vi "AK Amium Auswerten.vi"(8 "Verknüpfter String":string, 9 "ATEM Index":string[](array[string]), 10 "Array":string[](array[string])) -> ()   [LabVIEW 2020, in "Amium PNS.lvlib" / "AK Kommunikation.lvlib"]
uses:
  AK Kommunikation.lvlib
  Aktion FGV Amium Daten.ctl
  Amium Kommandos verwalten Aktionen.ctl
  Amium Zustand.ctl
  Amium ErrorCluster.ctl
  Amium PNS.lvlib
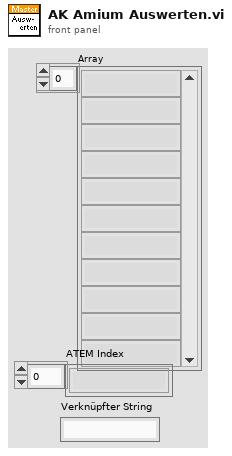
[diagram p1: front panel]
types:
  T1 = typedef "Amium PNS.lvlib/Aktion FGV Amium Daten.ctl" = enum16{"lesen", "Komm Daten", "Daten", "Error", "Regler", "Grenzwerte", "laden", "speichern"}
  T2 = typedef "Amium PNS.lvlib/AK Kommunikation.lvlib/Amium Kommandos verwalten Aktionen.ctl" = enum16{"lesen", "setzen Ende", "setzen Pos1", "senden", "initalisieren", "prüfen", "Kommandos"}
  T3 = typedef "Amium PNS.lvlib/Amium ErrorCluster.ctl" = cluster{"Messgasdruck":bool, "Temperatur":bool, "Steuerluft":bool, "Temperatur HL 1":bool, "Temperatur HL 2":bool, "Temperatur HL 3":bool, "Temperatur HL 4":bool, "Temperatur HL 5":bool, "Temperatur HL 6":bool, "Temperatur HL 7":bool, "Temperatur HL 8":bool, "Temperatur HL 9":bool, "Temperatur HL 10":bool, "Temperatur 11 Ofen MGF/Filter":bool, "Temperatur HL12":bool, "Temperatur 13 Ofen MGP/Pumpe":bool, "Temperatur HL 14":bool}
  T4 = typedef "Amium PNS.lvlib/Daten Cluster.ctl" = cluster{"Amium Zustände":T5, "Samplepoint am PNS":i16, "Gerätekennung":string, "aktiver Samplepoint":i16[], "Messgasdruck":sgl}
  T5 = typedef "Amium PNS.lvlib/Amium Zustand.ctl" = u16
  T6 = typedef "Amium PNS.lvlib/Temperaturregler Cluster.ctl" = cluster{"Istwert":sgl, "Sollwert":sgl, "Stellgröße":sgl, "Status":sgl, "Error":sgl}
  T7 = typedef "Amium PNS.lvlib/Amium Anlagengrenzwerte PNS.ctl" = cluster{"Filter:":T8, "Ventilplatte:":T8, "Heizleitung 1:":T8, "Heizleitung 2:":T8, "Heizleitung 3:":T8, "Heizleitung 4:":T8, "Heizleitung 5:":T8, "Heizleitung 6:":T8, "Heizleitung 7:":T8, "Heizleitung 8:":T8, "Heizleitung 9:":T8, "Heizleitung 10:":T8, "Heizleitung 11:":T8, "Heizleitung 12:":T8}
  T8 = typedef "Amium PNS.lvlib/Amium Anlagengrenzwerte-Parameter Anzeige.ctl" = cluster{"Sollwert":T9, "Warn-Min":T9, "Warn-Max":T9, "Abschalt-Min":T9, "Abschalt-Max":T9, "Regler":u16}
  T9 = typedef "Zahlen-Eingabefeld.ctl" = sgl
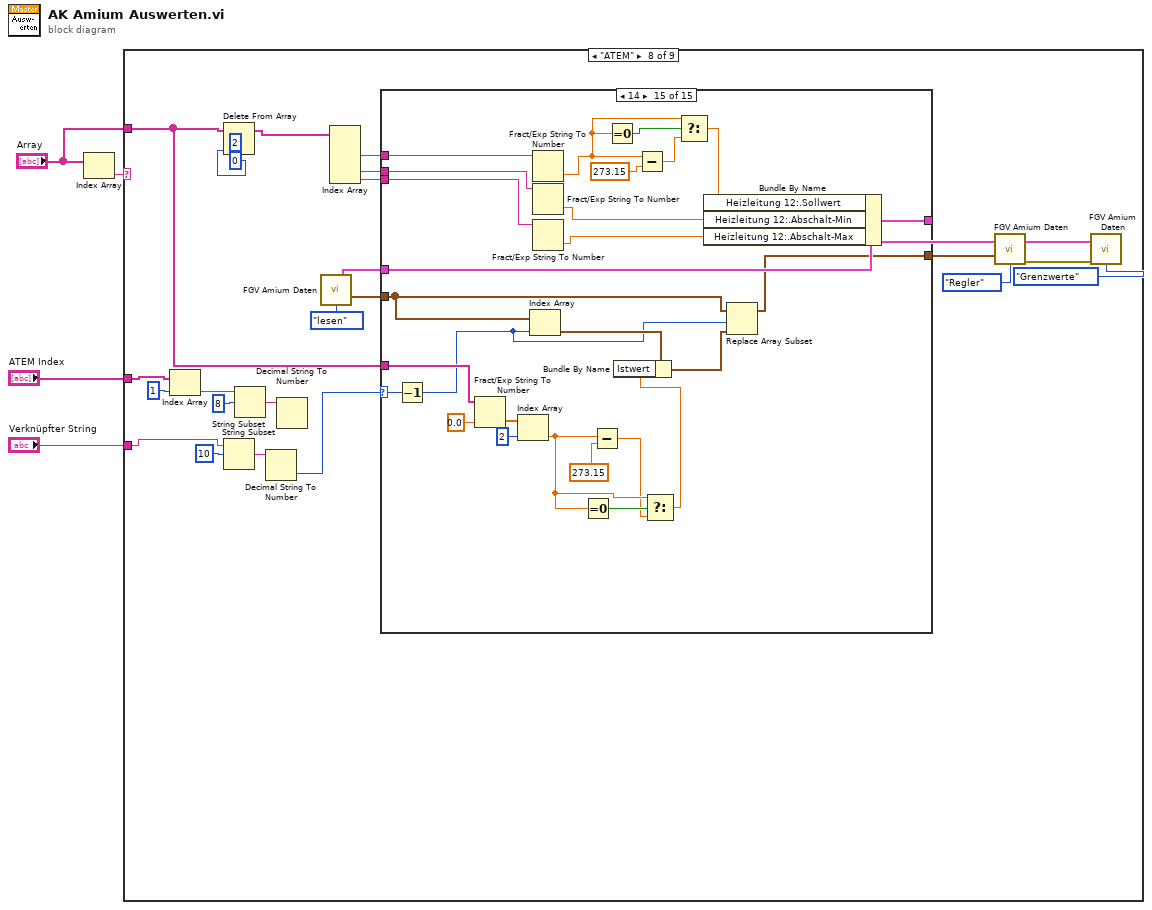
[diagram p0: block diagram]
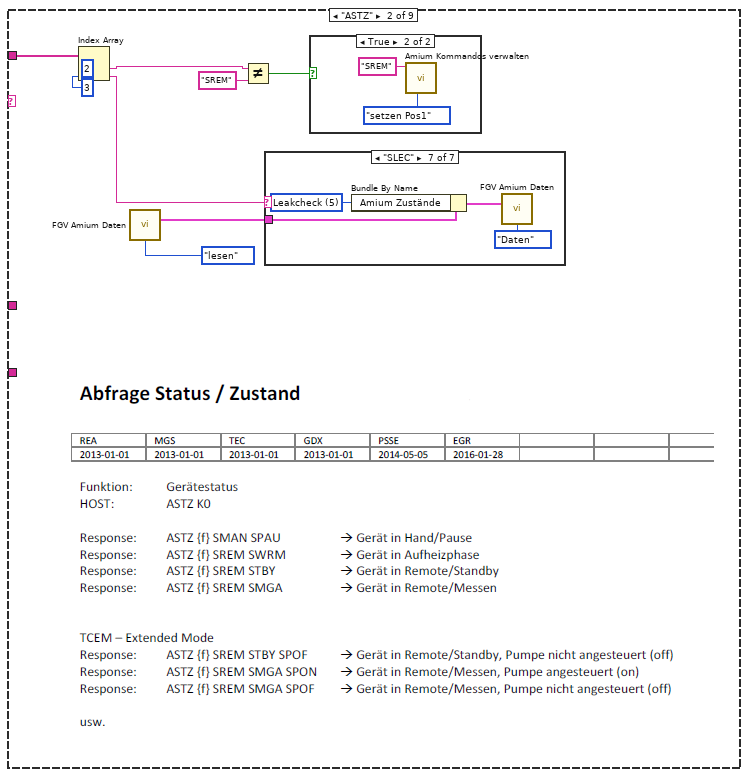
[diagram p3: hidden frame]
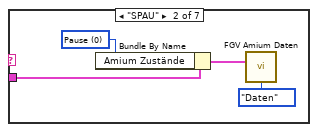
[diagram p5: hidden frame]
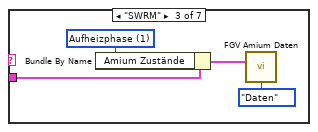
[diagram p6: hidden frame]
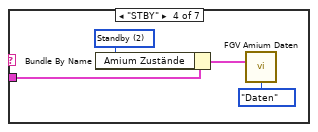
[diagram p7: hidden frame]
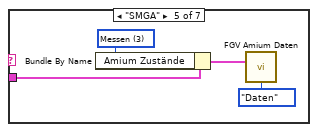
[diagram p8: hidden frame]
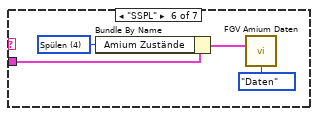
[diagram p9: hidden frame]
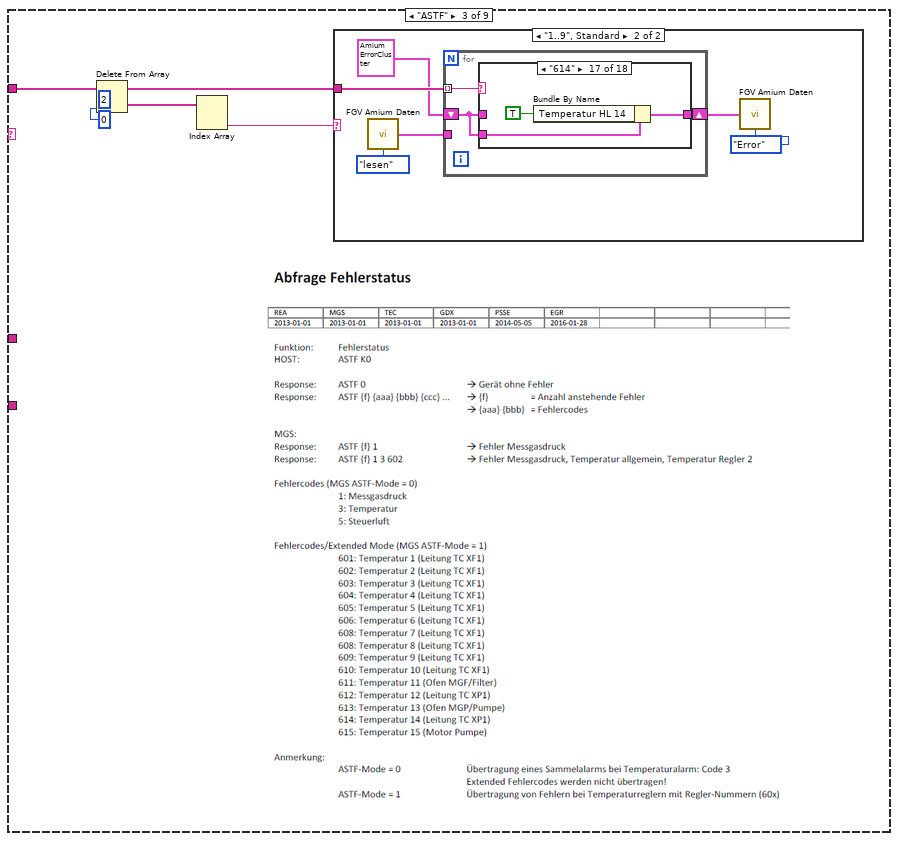
[diagram p11: hidden frame]
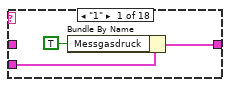
[diagram p13: hidden frame]
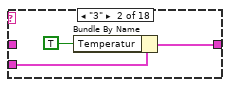
[diagram p14: hidden frame]
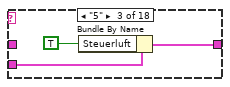
[diagram p15: hidden frame]
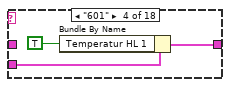
[diagram p16: hidden frame]
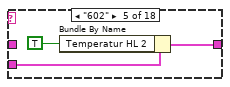
[diagram p17: hidden frame]
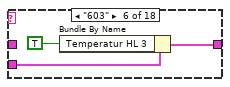
[diagram p18: hidden frame]
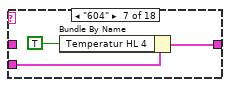
[diagram p19: hidden frame]
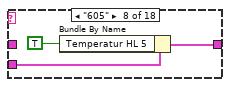
[diagram p20: hidden frame]
diagram:
  n1 = Index Array(array="Array") -> (element=w4:string)  [unwired: 1 in]
  n2 = case shown="\"ATEM\"" w4 {
    tunnel: "Array" -> [_ w13 w45 w115 w122 w136 w170 w180 w588]
    tunnel: "ATEM Index" -> [_ _ _ _ _ _ _ w185 _]
    tunnel: "Verknüpfter String" -> [_ _ _ _ _ w124 _ w184 _]
    frame "False", Default {
    }
    frame "ASTZ" {
      n3 = Index Array(array=w13, index #1=2 ("Index"), index #2=3 ("Index")) -> (element #1=w10:string, element #2=w7:string)
      n4 = call "FGV Amium Daten.vi"("Aktion"=Aktion_FGV_Amium_Daten."lesen") -> ("Amium Daten"=w5:T4)  [unwired: 9 in, 5 out]
      n5 = Not Equal?(x=w10, y="SREM" ("neues Kommando")) -> (x != y?=w9:bool)
      n6 = case shown="\"SLEC\"" w7 {
        tunnel: w5 -> [_ w17 w21 w25 w29 w33 w37]
        frame "False", Default {
        }
        frame "SPAU" {
          w16 = T5 0 items=["Pause", "Aufheizphase", "Standby", "Messen"] ("Amium Zustände")
          n7 = Bundle By Name(cluster=w17, "Amium Zustände"=w16) -> (w14:T4)
          n8 = call "FGV Amium Daten.vi"("Amium Daten"=w14, "Aktion"=Aktion_FGV_Amium_Daten."Daten") -> ()  [unwired: 8 in, 6 out]
        }
        frame "SWRM" {
          w20 = T5 1 items=["Pause", "Aufheizphase", "Standby", "Messen"] ("Amium Zustände")
          n9 = Bundle By Name(cluster=w21, "Amium Zustände"=w20) -> (w18:T4)
          n10 = call "FGV Amium Daten.vi"("Amium Daten"=w18, "Aktion"=Aktion_FGV_Amium_Daten."Daten") -> ()  [unwired: 8 in, 6 out]
        }
        frame "STBY" {
          w24 = T5 2 items=["Pause", "Aufheizphase", "Standby", "Messen"] ("Amium Zustände")
          n11 = Bundle By Name(cluster=w25, "Amium Zustände"=w24) -> (w22:T4)
          n12 = call "FGV Amium Daten.vi"("Amium Daten"=w22, "Aktion"=Aktion_FGV_Amium_Daten."Daten") -> ()  [unwired: 8 in, 6 out]
        }
        frame "SMGA" {
          w28 = T5 3 items=["Pause", "Aufheizphase", "Standby", "Messen"] ("Amium Zustände")
          n13 = Bundle By Name(cluster=w29, "Amium Zustände"=w28) -> (w26:T4)
          n14 = call "FGV Amium Daten.vi"("Amium Daten"=w26, "Aktion"=Aktion_FGV_Amium_Daten."Daten") -> ()  [unwired: 8 in, 6 out]
        }
        frame "SSPL" {
          w30 = T5 4 items=["Pause", "Aufheizphase", "Standby", "Messen", "Spülen"] ("Amium Zustände")
          n15 = Bundle By Name(cluster=w33, "Amium Zustände"=w30) -> (w31:T4)
          n16 = call "FGV Amium Daten.vi"("Amium Daten"=w31, "Aktion"=Aktion_FGV_Amium_Daten."Daten") -> ()  [unwired: 8 in, 6 out]
        }
        frame "SLEC" {
          w34 = T5 5 items=["Pause", "Aufheizphase", "Standby", "Messen", "Spülen", "Leakcheck"] ("Amium Zustände")
          n17 = Bundle By Name(cluster=w37, "Amium Zustände"=w34) -> (w35:T4)
          n18 = call "FGV Amium Daten.vi"("Amium Daten"=w35, "Aktion"=Aktion_FGV_Amium_Daten."Daten") -> ()  [unwired: 8 in, 6 out]
        }
      }
      n19 = case shown="True" w9 {
        frame False {
        }
        frame True {
          n20 = call "Amium Kommandos verwalten.vi"("Aktionen"=Amium_Kommandos_verwalten_Aktionen."setzen Pos1", "neues Kommando"="SREM") -> ()  [unwired: 7 in, 3 out]
        }
      }
    }
    frame "ASTF" {
      n21 = Delete From Array(array=w45, length=2 ("Länge"), index=0 ("Index")) -> (deleted portion=w41:string[], array with subset deleted=w42:string[])
      n22 = Index Array(array=w41) -> (element #2=w40:string)  [unwired: 2 in, 1 out]
      n23 = case shown="\"1..9\", Standard" w40 {
        tunnel: w42 -> [_ w51]
        frame "0" {
        }
        frame "1..9", Default {
          n24 = call "FGV Amium Daten.vi"("Aktion"=Aktion_FGV_Amium_Daten."lesen") -> ("Fehler Cluster"=w47:T3)  [unwired: 9 in, 5 out]
          n25 = for {
            tunnel: w51 -> [w54] mode=indexing
            shift-right: [w53] -> w48
            shift-left: T3 {"Messgasdruck"=FALSE, "Temperatur"=FALSE, "Steuerluft"=FALSE, "Temperatur HL 1"=FALSE, "Temperatur HL 2"=FALSE, "Temperatur HL 3"=FALSE, "Temperatur HL 4"=FALSE, "Temperatur HL 5"=FALSE, "Temperatur HL 6"=FALSE, "Temperatur HL 7"=FALSE, "Temperatur HL 8"=FALSE, "Temperatur HL 9"=FALSE, "Temperatur HL 10"=FALSE, "Temperatur 11 Ofen MGF/Filter"=FALSE, "Temperatur HL12"=FALSE, "Temperatur 13 Ofen MGP/Pumpe"=FALSE, "Temperatur HL 14"=FALSE} ("Fehler Cluster") -> [w52]
            tunnel: w47 -> [_]
            n26 = case shown="\"614\"" w54 {
              tunnel: w52 -> [w57 w60 w63 w66 w69 w72 w75 w78 w81 w84 w87 w90 w93 w96 w99 w102 w105 _]
              tunnel: [w55 w58 w61 w64 w67 w70 w73 w76 w79 w82 w85 w88 w91 w94 w97 w100 w103 w106] -> w53
              tunnel: w52 -> [_ _ _ _ _ _ _ _ _ _ _ _ _ _ _ _ _ w106]
              frame "1" {
                n27 = Bundle By Name(cluster=w57, "Messgasdruck"=TRUE) -> (w55:T3)
              }
              frame "3" {
                n28 = Bundle By Name(cluster=w60, "Temperatur"=TRUE ("Messgasdruck")) -> (w58:T3)
              }
              frame "5" {
                n29 = Bundle By Name(cluster=w63, "Steuerluft"=TRUE ("Messgasdruck")) -> (w61:T3)
              }
              frame "601" {
                n30 = Bundle By Name(cluster=w66, "Temperatur HL 1"=TRUE ("Messgasdruck")) -> (w64:T3)
              }
              frame "602" {
                n31 = Bundle By Name(cluster=w69, "Temperatur HL 2"=TRUE ("Messgasdruck")) -> (w67:T3)
              }
              frame "603" {
                n32 = Bundle By Name(cluster=w72, "Temperatur HL 3"=TRUE ("Messgasdruck")) -> (w70:T3)
              }
              frame "604" {
                n33 = Bundle By Name(cluster=w75, "Temperatur HL 4"=TRUE ("Messgasdruck")) -> (w73:T3)
              }
              frame "605" {
                n34 = Bundle By Name(cluster=w78, "Temperatur HL 5"=TRUE ("Messgasdruck")) -> (w76:T3)
              }
              frame "606" {
                n35 = Bundle By Name(cluster=w81, "Temperatur HL 6"=TRUE ("Messgasdruck")) -> (w79:T3)
              }
              frame "607" {
                n36 = Bundle By Name(cluster=w84, "Temperatur HL 7"=TRUE ("Messgasdruck")) -> (w82:T3)
              }
              frame "608" {
                n37 = Bundle By Name(cluster=w87, "Temperatur HL 8"=TRUE ("Messgasdruck")) -> (w85:T3)
              }
              frame "609" {
                n38 = Bundle By Name(cluster=w90, "Temperatur HL 9"=TRUE ("Messgasdruck")) -> (w88:T3)
              }
              frame "610" {
                n39 = Bundle By Name(cluster=w93, "Temperatur HL 10"=TRUE ("Messgasdruck")) -> (w91:T3)
              }
              frame "611" {
                n40 = Bundle By Name(cluster=w96, "Temperatur 11 Ofen MGF/Filter"=TRUE ("Messgasdruck")) -> (w94:T3)
              }
              frame "612" {
                n41 = Bundle By Name(cluster=w99, "Temperatur HL12"=TRUE ("Messgasdruck")) -> (w97:T3)
              }
              frame "613" {
                n42 = Bundle By Name(cluster=w102, "Temperatur 13 Ofen MGP/Pumpe"=TRUE ("Messgasdruck")) -> (w100:T3)
              }
              frame "614" {
                n43 = Bundle By Name(cluster=w105, "Temperatur HL 14"=TRUE ("Messgasdruck")) -> (w103:T3)
              }
              frame "0", Default {
              }
            }
          }
          n44 = call "FGV Amium Daten.vi"("Fehler Cluster"=w48, "Aktion"=Aktion_FGV_Amium_Daten."Error") -> ()  [unwired: 8 in, 6 out]
        }
      }
    }
    frame "ACFG" {
      n45 = Index Array(array=w115, index=2 ("Index")) -> (element=w113:string)
      n46 = Decimal String To Number(string=w113, default (0L)=i16 0 ("Samplepoint am PNS")) -> (number=w110:i16)  [unwired: 1 in, 1 out]
      n47 = call "FGV Amium Daten.vi"("Aktion"=Aktion_FGV_Amium_Daten."lesen") -> ("Amium Daten"=w111:T4)  [unwired: 9 in, 5 out]
      n48 = Bundle By Name(cluster=w111, "Samplepoint am PNS"=w110) -> (w107:T4)
      n49 = call "FGV Amium Daten.vi"("Amium Daten"=w107, "Aktion"=Aktion_FGV_Amium_Daten."Daten") -> ()  [unwired: 8 in, 6 out]
    }
    frame "AKEN" {
      n50 = Index Array(array=w122, index=2 ("Index")) -> (element=w116:string)
      n51 = call "FGV Amium Daten.vi"("Aktion"=Aktion_FGV_Amium_Daten."lesen") -> ("Amium Daten"=w119:T4)  [unwired: 9 in, 5 out]
      n52 = Bundle By Name(cluster=w119, "Gerätekennung"=w116) -> (w117:T4)
      n53 = call "FGV Amium Daten.vi"("Amium Daten"=w117, "Aktion"=Aktion_FGV_Amium_Daten."Daten") -> ()  [unwired: 8 in, 6 out]
    }
    frame "ATES" {
      n54 = String Subset(string=w124, offset (0)=10 ("Offset (0)")) -> (substring=w126:string)  [unwired: 1 in]
      n55 = Delete From Array(array=w136, length=2 ("Länge"), index=0 ("Index")) -> (array with subset deleted=w131:string[])  [unwired: 1 out]
      n56 = Decimal String To Number(string=w126) -> (number=w123:i32)  [unwired: 2 in, 1 out]
      n57 = Array Size(array=w131) -> (size(s)=w130:i32)
      n58 = Fract/Exp String To Number(string=w131, default (0 dbl)=sgl 0.0) -> (number=w132:sgl[])  [unwired: 2 in, 1 out]
      n59 = To Double Precision Float(number=w130) -> (double precision float=w127:dbl)
      n60 = Divide(x=w127, y=5.0) -> (x/y=w128:dbl)
      n61 = To Long Integer(number=w128) -> ()  [unwired: 1 out]
      n62 = case shown="0..14, Standard" w123 {
        selector: w123 -> [_ w163]
        tunnel: w132 -> [w138 w154]
        frame 20 {
          n63 = for {
            N: 10 -> [_]
            shift-right: [w151] -> _
            shift-left: w138 -> [w152]
            tunnel: [w139] -> _
            i -> [w141]
            stop <- w150 stop-if-true
            n64 = Split 1D Array(array=w152, index=5 ("Index")) -> (first subarray=w148:sgl[], second subarray=w151:sgl[])
            n65 = Empty Array?(array=w151) -> (empty?=w150:bool)
            n66 = Index Array(array=w148, index=3 ("Index")) -> (element=w142:sgl)
            n67 = call "FGV Amium Daten.vi"("Aktion"=Aktion_FGV_Amium_Daten."lesen") -> ("Regler"=w145:T6[])  [unwired: 9 in, 5 out]
            n68 = Index Array(array=w145, index=w141) -> (element=w146:T6)
            n69 = Bundle By Name(cluster=w146, "Status"=w142) -> (w144:T6)
            n70 = Replace Array Subset(array=w145, new element=w144, index=w141) -> (w139:T6[])
            n71 = call "FGV Amium Daten.vi"("Regler"=w139, "Aktion"=Aktion_FGV_Amium_Daten."Regler") -> ()  [unwired: 8 in, 6 out]
          }
        }
        frame 0..14, Default {
          (unwired) 10
          n72 = Decrement(x=w163) -> (x-1=w153:i32)
          n73 = Index Array(array=w154, index=3 ("Index")) -> (element=w157:sgl)
          n74 = call "FGV Amium Daten.vi"("Aktion"=Aktion_FGV_Amium_Daten."lesen") -> ("Regler"=w160:T6[])  [unwired: 9 in, 5 out]
          n75 = Index Array(array=w160, index=w153) -> (element=w161:T6)
          n76 = Bundle By Name(cluster=w161, "Status"=w157) -> (w159:T6)
          n77 = Replace Array Subset(array=w160, new element=w159, index=w153) -> (w155:T6[])
          n78 = call "FGV Amium Daten.vi"("Regler"=w155, "Aktion"=Aktion_FGV_Amium_Daten."Regler") -> ()  [unwired: 8 in, 6 out]
        }
      }
    }
    frame "AENT" {
      n79 = Delete From Array(array=w170, length=2 ("Länge"), index=0 ("Index")) -> (array with subset deleted=w164:string[])  [unwired: 1 out]
      n80 = call "FGV Amium Daten.vi"("Aktion"=Aktion_FGV_Amium_Daten."lesen") -> ("Amium Daten"=w168:T4)  [unwired: 9 in, 5 out]
      n81 = for {
        tunnel: [w174] -> w167 mode=indexing
        tunnel: w164 -> [w173] mode=indexing
        n82 = Decimal String To Number(string=w173, default (0L)=i16 0 ("Samplepoint am PNS")) -> (number=w174:i16)  [unwired: 1 in, 1 out]
      }
      n83 = Bundle By Name(cluster=w168, "aktiver Samplepoint"=w167) -> (w165:T4)
      n84 = call "FGV Amium Daten.vi"("Amium Daten"=w165, "Aktion"=Aktion_FGV_Amium_Daten."Daten") -> ()  [unwired: 8 in, 6 out]
    }
    frame "ATEM" {
      n85 = Index Array(array=w185, index=1 ("Index")) -> (element=w187:string)
      n86 = Delete From Array(array=w180, length=2 ("Länge"), index=0 ("Index")) -> (array with subset deleted=w193:string[])  [unwired: 1 out]
      n87 = String Subset(string=w184, offset (0)=10 ("Offset (0)")) -> (substring=w183:string)  [unwired: 1 in]
      n88 = String Subset(string=w187, offset (0)=8 ("Offset (0)")) -> (substring=w194:string)  [unwired: 1 in]
      n89 = Decimal String To Number(string=w183) -> (number=w181:i32)  [unwired: 2 in, 1 out]
      n90 = Decimal String To Number(string=w194) -> ()  [unwired: 2 in, 2 out]
      n91 = call "FGV Amium Daten.vi"("Aktion"=Aktion_FGV_Amium_Daten."lesen") -> ("Grenzwerte PNS"=w196:T7, "Regler"=w176:T6[])  [unwired: 9 in, 4 out]
      n92 = Index Array(array=w193) -> (element #2=w192:string, element #4=w191:string, element #5=w190:string)  [unwired: 5 in, 2 out]
      n93 = case shown="14" w181 {
        selector: w181 -> [_ w219 w246 w273 w300 w327 w354 w381 w408 w435 w462 w489 w516 w543 w570]
        tunnel: w196 -> [w201 w228 w255 w282 w309 w336 w363 w390 w417 w444 w471 w498 w525 w552 w579]
        tunnel: w192 -> [_ w227 w254 w281 w308 w335 w362 w389 w416 w443 w470 w497 w524 w551 w578]
        tunnel: w191 -> [_ w226 w253 w280 w307 w334 w361 w388 w415 w442 w469 w496 w523 w550 w577]
        tunnel: w190 -> [_ w224 w251 w278 w305 w332 w359 w386 w413 w440 w467 w494 w521 w548 w575]
        tunnel: [w201 w222 w249 w276 w303 w330 w357 w384 w411 w438 w465 w492 w519 w546 w573] -> w188
        tunnel: w180 -> [_ w220 w247 w274 w301 w328 w355 w382 w409 w436 w463 w490 w517 w544 w571]
        tunnel: [w200 w212 w239 w266 w293 w320 w347 w374 w401 w428 w455 w482 w509 w536 w563] -> w178
        tunnel: w176 -> [w200 w214 w241 w268 w295 w322 w349 w376 w403 w430 w457 w484 w511 w538 w565]
        frame 0, Default {
        }
        frame 1 {
          n94 = Decrement(x=w219) -> (x-1=w213:i32)
          n95 = Fract/Exp String To Number(string=w220, default (0 dbl)=sgl 0.0) -> (number=w217:sgl[])  [unwired: 2 in, 1 out]
          n96 = Index Array(array=w217, index=2 ("Index")) -> (element=w204:sgl)
          n97 = Index Array(array=w214, index=w213) -> (element=w218:T6)
          n98 = Fract/Exp String To Number(string=w227) -> (number=w208:dbl)  [unwired: 3 in, 1 out]
          n99 = Fract/Exp String To Number(string=w226) -> (number=w225:dbl)  [unwired: 3 in, 1 out]
          n100 = Fract/Exp String To Number(string=w224) -> (number=w223:dbl)  [unwired: 3 in, 1 out]
          n101 = Equal To 0?(x=w204) -> (x = 0?=w205:bool)
          n102 = Subtract(x=w204, y=273.15) -> (x-y=w203:dbl)
          n103 = Equal To 0?(x=w208) -> (x = 0?=w207:bool)
          n104 = Subtract(x=w208, y=273.15) -> (x-y=w209:dbl)
          n105 = Select(t=w204, s=w205, f=w203) -> (s? t:f=w202:dbl)
          n106 = Bundle By Name(cluster=w218, "Istwert"=w202) -> (w215:T6)
          n107 = Select(t=w208, s=w207, f=w209) -> (s? t:f=w206:dbl)
          n108 = Bundle By Name(cluster=w228, "Filter:.Sollwert"=w206, "Filter:.Abschalt-Min"=w225, "Filter:.Abschalt-Max"=w223) -> (w222:T7)
          n109 = Replace Array Subset(array=w214, new element=w215, index=w213) -> (w212:T6[])
        }
        frame 2 {
          n110 = Decrement(x=w246) -> (x-1=w240:i32)
          n111 = Fract/Exp String To Number(string=w247, default (0 dbl)=sgl 0.0) -> (number=w244:sgl[])  [unwired: 2 in, 1 out]
          n112 = Index Array(array=w244, index=2 ("Index")) -> (element=w231:sgl)
          n113 = Index Array(array=w241, index=w240) -> (element=w245:T6)
          n114 = Fract/Exp String To Number(string=w254) -> (number=w235:dbl)  [unwired: 3 in, 1 out]
          n115 = Fract/Exp String To Number(string=w253) -> (number=w252:dbl)  [unwired: 3 in, 1 out]
          n116 = Fract/Exp String To Number(string=w251) -> (number=w250:dbl)  [unwired: 3 in, 1 out]
          n117 = Equal To 0?(x=w231) -> (x = 0?=w232:bool)
          n118 = Subtract(x=w231, y=273.15) -> (x-y=w230:dbl)
          n119 = Equal To 0?(x=w235) -> (x = 0?=w234:bool)
          n120 = Subtract(x=w235, y=273.15) -> (x-y=w236:dbl)
          n121 = Select(t=w231, s=w232, f=w230) -> (s? t:f=w229:dbl)
          n122 = Bundle By Name(cluster=w245, "Istwert"=w229) -> (w242:T6)
          n123 = Select(t=w235, s=w234, f=w236) -> (s? t:f=w233:dbl)
          n124 = Bundle By Name(cluster=w255, "Ventilplatte:.Sollwert"=w233, "Ventilplatte:.Abschalt-Min"=w252, "Ventilplatte:.Abschalt-Max"=w250) -> (w249:T7)
          n125 = Replace Array Subset(array=w241, new element=w242, index=w240) -> (w239:T6[])
        }
        frame 3 {
          n126 = Decrement(x=w273) -> (x-1=w267:i32)
          n127 = Fract/Exp String To Number(string=w274, default (0 dbl)=sgl 0.0) -> (number=w271:sgl[])  [unwired: 2 in, 1 out]
          n128 = Index Array(array=w271, index=2 ("Index")) -> (element=w258:sgl)
          n129 = Index Array(array=w268, index=w267) -> (element=w272:T6)
          n130 = Fract/Exp String To Number(string=w281) -> (number=w262:dbl)  [unwired: 3 in, 1 out]
          n131 = Fract/Exp String To Number(string=w280) -> (number=w279:dbl)  [unwired: 3 in, 1 out]
          n132 = Fract/Exp String To Number(string=w278) -> (number=w277:dbl)  [unwired: 3 in, 1 out]
          n133 = Equal To 0?(x=w258) -> (x = 0?=w259:bool)
          n134 = Subtract(x=w258, y=273.15) -> (x-y=w257:dbl)
          n135 = Equal To 0?(x=w262) -> (x = 0?=w261:bool)
          n136 = Subtract(x=w262, y=273.15) -> (x-y=w263:dbl)
          n137 = Select(t=w258, s=w259, f=w257) -> (s? t:f=w256:dbl)
          n138 = Bundle By Name(cluster=w272, "Istwert"=w256) -> (w269:T6)
          n139 = Select(t=w262, s=w261, f=w263) -> (s? t:f=w260:dbl)
          n140 = Bundle By Name(cluster=w282, "Heizleitung 1:.Sollwert"=w260, "Heizleitung 1:.Abschalt-Min"=w279, "Heizleitung 1:.Abschalt-Max"=w277) -> (w276:T7)
          n141 = Replace Array Subset(array=w268, new element=w269, index=w267) -> (w266:T6[])
        }
        frame 4 {
          n142 = Decrement(x=w300) -> (x-1=w294:i32)
          n143 = Fract/Exp String To Number(string=w301, default (0 dbl)=sgl 0.0) -> (number=w298:sgl[])  [unwired: 2 in, 1 out]
          n144 = Index Array(array=w298, index=2 ("Index")) -> (element=w285:sgl)
          n145 = Index Array(array=w295, index=w294) -> (element=w299:T6)
          n146 = Fract/Exp String To Number(string=w308) -> (number=w289:dbl)  [unwired: 3 in, 1 out]
          n147 = Fract/Exp String To Number(string=w307) -> (number=w306:dbl)  [unwired: 3 in, 1 out]
          n148 = Fract/Exp String To Number(string=w305) -> (number=w304:dbl)  [unwired: 3 in, 1 out]
          n149 = Equal To 0?(x=w285) -> (x = 0?=w286:bool)
          n150 = Subtract(x=w285, y=273.15) -> (x-y=w284:dbl)
          n151 = Equal To 0?(x=w289) -> (x = 0?=w288:bool)
          n152 = Subtract(x=w289, y=273.15) -> (x-y=w290:dbl)
          n153 = Select(t=w285, s=w286, f=w284) -> (s? t:f=w283:dbl)
          n154 = Bundle By Name(cluster=w299, "Istwert"=w283) -> (w296:T6)
          n155 = Select(t=w289, s=w288, f=w290) -> (s? t:f=w287:dbl)
          n156 = Bundle By Name(cluster=w309, "Heizleitung 2:.Sollwert"=w287, "Heizleitung 2:.Abschalt-Min"=w306, "Heizleitung 2:.Abschalt-Max"=w304) -> (w303:T7)
          n157 = Replace Array Subset(array=w295, new element=w296, index=w294) -> (w293:T6[])
        }
        frame 5 {
          n158 = Decrement(x=w327) -> (x-1=w321:i32)
          n159 = Fract/Exp String To Number(string=w328, default (0 dbl)=sgl 0.0) -> (number=w325:sgl[])  [unwired: 2 in, 1 out]
          n160 = Index Array(array=w325, index=2 ("Index")) -> (element=w312:sgl)
          n161 = Index Array(array=w322, index=w321) -> (element=w326:T6)
          n162 = Fract/Exp String To Number(string=w335) -> (number=w316:dbl)  [unwired: 3 in, 1 out]
          n163 = Fract/Exp String To Number(string=w334) -> (number=w333:dbl)  [unwired: 3 in, 1 out]
          n164 = Fract/Exp String To Number(string=w332) -> (number=w331:dbl)  [unwired: 3 in, 1 out]
          n165 = Equal To 0?(x=w312) -> (x = 0?=w313:bool)
          n166 = Subtract(x=w312, y=273.15) -> (x-y=w311:dbl)
          n167 = Equal To 0?(x=w316) -> (x = 0?=w315:bool)
          n168 = Subtract(x=w316, y=273.15) -> (x-y=w317:dbl)
          n169 = Select(t=w312, s=w313, f=w311) -> (s? t:f=w310:dbl)
          n170 = Bundle By Name(cluster=w326, "Istwert"=w310) -> (w323:T6)
          n171 = Select(t=w316, s=w315, f=w317) -> (s? t:f=w314:dbl)
          n172 = Bundle By Name(cluster=w336, "Heizleitung 3:.Sollwert"=w314, "Heizleitung 3:.Abschalt-Min"=w333, "Heizleitung 3:.Abschalt-Max"=w331) -> (w330:T7)
          n173 = Replace Array Subset(array=w322, new element=w323, index=w321) -> (w320:T6[])
        }
        frame 6 {
          n174 = Decrement(x=w354) -> (x-1=w348:i32)
          n175 = Fract/Exp String To Number(string=w355, default (0 dbl)=sgl 0.0) -> (number=w352:sgl[])  [unwired: 2 in, 1 out]
          n176 = Index Array(array=w352, index=2 ("Index")) -> (element=w339:sgl)
          n177 = Index Array(array=w349, index=w348) -> (element=w353:T6)
          n178 = Fract/Exp String To Number(string=w362) -> (number=w343:dbl)  [unwired: 3 in, 1 out]
          n179 = Fract/Exp String To Number(string=w361) -> (number=w360:dbl)  [unwired: 3 in, 1 out]
          n180 = Fract/Exp String To Number(string=w359) -> (number=w358:dbl)  [unwired: 3 in, 1 out]
          n181 = Equal To 0?(x=w339) -> (x = 0?=w340:bool)
          n182 = Subtract(x=w339, y=273.15) -> (x-y=w338:dbl)
          n183 = Equal To 0?(x=w343) -> (x = 0?=w342:bool)
          n184 = Subtract(x=w343, y=273.15) -> (x-y=w344:dbl)
          n185 = Select(t=w339, s=w340, f=w338) -> (s? t:f=w337:dbl)
          n186 = Bundle By Name(cluster=w353, "Istwert"=w337) -> (w350:T6)
          n187 = Select(t=w343, s=w342, f=w344) -> (s? t:f=w341:dbl)
          n188 = Bundle By Name(cluster=w363, "Heizleitung 4:.Sollwert"=w341, "Heizleitung 4:.Abschalt-Min"=w360, "Heizleitung 4:.Abschalt-Max"=w358) -> (w357:T7)
          n189 = Replace Array Subset(array=w349, new element=w350, index=w348) -> (w347:T6[])
        }
        frame 7 {
          n190 = Decrement(x=w381) -> (x-1=w375:i32)
          n191 = Fract/Exp String To Number(string=w382, default (0 dbl)=sgl 0.0) -> (number=w379:sgl[])  [unwired: 2 in, 1 out]
          n192 = Index Array(array=w379, index=2 ("Index")) -> (element=w366:sgl)
          n193 = Index Array(array=w376, index=w375) -> (element=w380:T6)
          n194 = Fract/Exp String To Number(string=w389) -> (number=w370:dbl)  [unwired: 3 in, 1 out]
          n195 = Fract/Exp String To Number(string=w388) -> (number=w387:dbl)  [unwired: 3 in, 1 out]
          n196 = Fract/Exp String To Number(string=w386) -> (number=w385:dbl)  [unwired: 3 in, 1 out]
          n197 = Equal To 0?(x=w366) -> (x = 0?=w367:bool)
          n198 = Subtract(x=w366, y=273.15) -> (x-y=w365:dbl)
          n199 = Equal To 0?(x=w370) -> (x = 0?=w369:bool)
          n200 = Subtract(x=w370, y=273.15) -> (x-y=w371:dbl)
          n201 = Select(t=w366, s=w367, f=w365) -> (s? t:f=w364:dbl)
          n202 = Bundle By Name(cluster=w380, "Istwert"=w364) -> (w377:T6)
          n203 = Select(t=w370, s=w369, f=w371) -> (s? t:f=w368:dbl)
          n204 = Bundle By Name(cluster=w390, "Heizleitung 5:.Sollwert"=w368, "Heizleitung 5:.Abschalt-Min"=w387, "Heizleitung 5:.Abschalt-Max"=w385) -> (w384:T7)
          n205 = Replace Array Subset(array=w376, new element=w377, index=w375) -> (w374:T6[])
        }
        frame 8 {
          n206 = Decrement(x=w408) -> (x-1=w402:i32)
          n207 = Fract/Exp String To Number(string=w409, default (0 dbl)=sgl 0.0) -> (number=w406:sgl[])  [unwired: 2 in, 1 out]
          n208 = Index Array(array=w406, index=2 ("Index")) -> (element=w393:sgl)
          n209 = Index Array(array=w403, index=w402) -> (element=w407:T6)
          n210 = Fract/Exp String To Number(string=w416) -> (number=w397:dbl)  [unwired: 3 in, 1 out]
          n211 = Fract/Exp String To Number(string=w415) -> (number=w414:dbl)  [unwired: 3 in, 1 out]
          n212 = Fract/Exp String To Number(string=w413) -> (number=w412:dbl)  [unwired: 3 in, 1 out]
          n213 = Equal To 0?(x=w393) -> (x = 0?=w394:bool)
          n214 = Subtract(x=w393, y=273.15) -> (x-y=w392:dbl)
          n215 = Equal To 0?(x=w397) -> (x = 0?=w396:bool)
          n216 = Subtract(x=w397, y=273.15) -> (x-y=w398:dbl)
          n217 = Select(t=w393, s=w394, f=w392) -> (s? t:f=w391:dbl)
          n218 = Bundle By Name(cluster=w407, "Istwert"=w391) -> (w404:T6)
          n219 = Select(t=w397, s=w396, f=w398) -> (s? t:f=w395:dbl)
          n220 = Bundle By Name(cluster=w417, "Heizleitung 6:.Sollwert"=w395, "Heizleitung 6:.Abschalt-Min"=w414, "Heizleitung 6:.Abschalt-Max"=w412) -> (w411:T7)
          n221 = Replace Array Subset(array=w403, new element=w404, index=w402) -> (w401:T6[])
        }
        frame 9 {
          n222 = Decrement(x=w435) -> (x-1=w429:i32)
          n223 = Fract/Exp String To Number(string=w436, default (0 dbl)=sgl 0.0) -> (number=w433:sgl[])  [unwired: 2 in, 1 out]
          n224 = Index Array(array=w433, index=2 ("Index")) -> (element=w420:sgl)
          n225 = Index Array(array=w430, index=w429) -> (element=w434:T6)
          n226 = Fract/Exp String To Number(string=w443) -> (number=w424:dbl)  [unwired: 3 in, 1 out]
          n227 = Fract/Exp String To Number(string=w442) -> (number=w441:dbl)  [unwired: 3 in, 1 out]
          n228 = Fract/Exp String To Number(string=w440) -> (number=w439:dbl)  [unwired: 3 in, 1 out]
          n229 = Equal To 0?(x=w420) -> (x = 0?=w421:bool)
          n230 = Subtract(x=w420, y=273.15) -> (x-y=w419:dbl)
          n231 = Equal To 0?(x=w424) -> (x = 0?=w423:bool)
          n232 = Subtract(x=w424, y=273.15) -> (x-y=w425:dbl)
          n233 = Select(t=w420, s=w421, f=w419) -> (s? t:f=w418:dbl)
          n234 = Bundle By Name(cluster=w434, "Istwert"=w418) -> (w431:T6)
          n235 = Select(t=w424, s=w423, f=w425) -> (s? t:f=w422:dbl)
          n236 = Bundle By Name(cluster=w444, "Heizleitung 7:.Sollwert"=w422, "Heizleitung 7:.Abschalt-Min"=w441, "Heizleitung 7:.Abschalt-Max"=w439) -> (w438:T7)
          n237 = Replace Array Subset(array=w430, new element=w431, index=w429) -> (w428:T6[])
        }
        frame 10 {
          n238 = Decrement(x=w462) -> (x-1=w456:i32)
          n239 = Fract/Exp String To Number(string=w463, default (0 dbl)=sgl 0.0) -> (number=w460:sgl[])  [unwired: 2 in, 1 out]
          n240 = Index Array(array=w460, index=2 ("Index")) -> (element=w447:sgl)
          n241 = Index Array(array=w457, index=w456) -> (element=w461:T6)
          n242 = Fract/Exp String To Number(string=w470) -> (number=w451:dbl)  [unwired: 3 in, 1 out]
          n243 = Fract/Exp String To Number(string=w469) -> (number=w468:dbl)  [unwired: 3 in, 1 out]
          n244 = Fract/Exp String To Number(string=w467) -> (number=w466:dbl)  [unwired: 3 in, 1 out]
          n245 = Equal To 0?(x=w447) -> (x = 0?=w448:bool)
          n246 = Subtract(x=w447, y=273.15) -> (x-y=w446:dbl)
          n247 = Equal To 0?(x=w451) -> (x = 0?=w450:bool)
          n248 = Subtract(x=w451, y=273.15) -> (x-y=w452:dbl)
          n249 = Select(t=w447, s=w448, f=w446) -> (s? t:f=w445:dbl)
          n250 = Bundle By Name(cluster=w461, "Istwert"=w445) -> (w458:T6)
          n251 = Select(t=w451, s=w450, f=w452) -> (s? t:f=w449:dbl)
          n252 = Bundle By Name(cluster=w471, "Heizleitung 8:.Sollwert"=w449, "Heizleitung 8:.Abschalt-Min"=w468, "Heizleitung 8:.Abschalt-Max"=w466) -> (w465:T7)
          n253 = Replace Array Subset(array=w457, new element=w458, index=w456) -> (w455:T6[])
        }
        frame 11 {
          n254 = Decrement(x=w489) -> (x-1=w483:i32)
          n255 = Fract/Exp String To Number(string=w490, default (0 dbl)=sgl 0.0) -> (number=w487:sgl[])  [unwired: 2 in, 1 out]
          n256 = Index Array(array=w487, index=2 ("Index")) -> (element=w474:sgl)
          n257 = Index Array(array=w484, index=w483) -> (element=w488:T6)
          n258 = Fract/Exp String To Number(string=w497) -> (number=w478:dbl)  [unwired: 3 in, 1 out]
          n259 = Fract/Exp String To Number(string=w496) -> (number=w495:dbl)  [unwired: 3 in, 1 out]
          n260 = Fract/Exp String To Number(string=w494) -> (number=w493:dbl)  [unwired: 3 in, 1 out]
          n261 = Equal To 0?(x=w474) -> (x = 0?=w475:bool)
          n262 = Subtract(x=w474, y=273.15) -> (x-y=w473:dbl)
          n263 = Equal To 0?(x=w478) -> (x = 0?=w477:bool)
          n264 = Subtract(x=w478, y=273.15) -> (x-y=w479:dbl)
          n265 = Select(t=w474, s=w475, f=w473) -> (s? t:f=w472:dbl)
          n266 = Bundle By Name(cluster=w488, "Istwert"=w472) -> (w485:T6)
          n267 = Select(t=w478, s=w477, f=w479) -> (s? t:f=w476:dbl)
          n268 = Bundle By Name(cluster=w498, "Heizleitung 9:.Sollwert"=w476, "Heizleitung 9:.Abschalt-Min"=w495, "Heizleitung 9:.Abschalt-Max"=w493) -> (w492:T7)
          n269 = Replace Array Subset(array=w484, new element=w485, index=w483) -> (w482:T6[])
        }
        frame 12 {
          n270 = Decrement(x=w516) -> (x-1=w510:i32)
          n271 = Fract/Exp String To Number(string=w517, default (0 dbl)=sgl 0.0) -> (number=w514:sgl[])  [unwired: 2 in, 1 out]
          n272 = Index Array(array=w514, index=2 ("Index")) -> (element=w501:sgl)
          n273 = Index Array(array=w511, index=w510) -> (element=w515:T6)
          n274 = Fract/Exp String To Number(string=w524) -> (number=w505:dbl)  [unwired: 3 in, 1 out]
          n275 = Fract/Exp String To Number(string=w523) -> (number=w522:dbl)  [unwired: 3 in, 1 out]
          n276 = Fract/Exp String To Number(string=w521) -> (number=w520:dbl)  [unwired: 3 in, 1 out]
          n277 = Equal To 0?(x=w501) -> (x = 0?=w502:bool)
          n278 = Subtract(x=w501, y=273.15) -> (x-y=w500:dbl)
          n279 = Equal To 0?(x=w505) -> (x = 0?=w504:bool)
          n280 = Subtract(x=w505, y=273.15) -> (x-y=w506:dbl)
          n281 = Select(t=w501, s=w502, f=w500) -> (s? t:f=w499:dbl)
          n282 = Bundle By Name(cluster=w515, "Istwert"=w499) -> (w512:T6)
          n283 = Select(t=w505, s=w504, f=w506) -> (s? t:f=w503:dbl)
          n284 = Bundle By Name(cluster=w525, "Heizleitung 10:.Sollwert"=w503, "Heizleitung 10:.Abschalt-Min"=w522, "Heizleitung 10:.Abschalt-Max"=w520) -> (w519:T7)
          n285 = Replace Array Subset(array=w511, new element=w512, index=w510) -> (w509:T6[])
        }
        frame 13 {
          n286 = Decrement(x=w543) -> (x-1=w537:i32)
          n287 = Fract/Exp String To Number(string=w544, default (0 dbl)=sgl 0.0) -> (number=w541:sgl[])  [unwired: 2 in, 1 out]
          n288 = Index Array(array=w541, index=2 ("Index")) -> (element=w528:sgl)
          n289 = Index Array(array=w538, index=w537) -> (element=w542:T6)
          n290 = Fract/Exp String To Number(string=w551) -> (number=w532:dbl)  [unwired: 3 in, 1 out]
          n291 = Fract/Exp String To Number(string=w550) -> (number=w549:dbl)  [unwired: 3 in, 1 out]
          n292 = Fract/Exp String To Number(string=w548) -> (number=w547:dbl)  [unwired: 3 in, 1 out]
          n293 = Equal To 0?(x=w528) -> (x = 0?=w529:bool)
          n294 = Subtract(x=w528, y=273.15) -> (x-y=w527:dbl)
          n295 = Equal To 0?(x=w532) -> (x = 0?=w531:bool)
          n296 = Subtract(x=w532, y=273.15) -> (x-y=w533:dbl)
          n297 = Select(t=w528, s=w529, f=w527) -> (s? t:f=w526:dbl)
          n298 = Bundle By Name(cluster=w542, "Istwert"=w526) -> (w539:T6)
          n299 = Select(t=w532, s=w531, f=w533) -> (s? t:f=w530:dbl)
          n300 = Bundle By Name(cluster=w552, "Heizleitung 11:.Sollwert"=w530, "Heizleitung 11:.Abschalt-Min"=w549, "Heizleitung 11:.Abschalt-Max"=w547) -> (w546:T7)
          n301 = Replace Array Subset(array=w538, new element=w539, index=w537) -> (w536:T6[])
        }
        frame 14 {
          n302 = Decrement(x=w570) -> (x-1=w564:i32)
          n303 = Fract/Exp String To Number(string=w571, default (0 dbl)=sgl 0.0) -> (number=w568:sgl[])  [unwired: 2 in, 1 out]
          n304 = Index Array(array=w568, index=2 ("Index")) -> (element=w555:sgl)
          n305 = Index Array(array=w565, index=w564) -> (element=w569:T6)
          n306 = Fract/Exp String To Number(string=w578) -> (number=w559:dbl)  [unwired: 3 in, 1 out]
          n307 = Fract/Exp String To Number(string=w577) -> (number=w576:dbl)  [unwired: 3 in, 1 out]
          n308 = Fract/Exp String To Number(string=w575) -> (number=w574:dbl)  [unwired: 3 in, 1 out]
          n309 = Equal To 0?(x=w555) -> (x = 0?=w556:bool)
          n310 = Subtract(x=w555, y=273.15) -> (x-y=w554:dbl)
          n311 = Equal To 0?(x=w559) -> (x = 0?=w558:bool)
          n312 = Subtract(x=w559, y=273.15) -> (x-y=w560:dbl)
          n313 = Select(t=w555, s=w556, f=w554) -> (s? t:f=w553:dbl)
          n314 = Bundle By Name(cluster=w569, "Istwert"=w553) -> (w566:T6)
          n315 = Select(t=w559, s=w558, f=w560) -> (s? t:f=w557:dbl)
          n316 = Bundle By Name(cluster=w579, "Heizleitung 12:.Sollwert"=w557, "Heizleitung 12:.Abschalt-Min"=w576, "Heizleitung 12:.Abschalt-Max"=w574) -> (w573:T7)
          n317 = Replace Array Subset(array=w565, new element=w566, index=w564) -> (w563:T6[])
        }
      }
      n318 = call "FGV Amium Daten.vi"("Regler"=w178, "Aktion"=Aktion_FGV_Amium_Daten."Regler") -> ("error out"=w177:errorcluster)  [unwired: 8 in, 5 out]
      n319 = call "FGV Amium Daten.vi"("Grenzwerte PNS"=w188, "error in (no error)"=w177, "Aktion"=Aktion_FGV_Amium_Daten."Grenzwerte") -> ()  [unwired: 7 in, 6 out]
    }
    frame "ADRU" {
      n320 = Index Array(array=w588) -> (element #3=w584:string)  [unwired: 3 in, 2 out]
      n321 = Fract/Exp String To Number(string=w584) -> (number=w581:dbl)  [unwired: 3 in, 1 out]
      n322 = call "FGV Amium Daten.vi"("Aktion"=Aktion_FGV_Amium_Daten."lesen") -> ("Amium Daten"=w585:T4)  [unwired: 9 in, 5 out]
      n323 = Divide(x=w581, y=1000.0) -> (x/y=w582:dbl)
      n324 = Bundle By Name(cluster=w585, "Messgasdruck"=w582) -> (w583:T4)
      n325 = call "FGV Amium Daten.vi"("Amium Daten"=w583, "Aktion"=Aktion_FGV_Amium_Daten."Daten") -> ()  [unwired: 8 in, 6 out]
    }
  }
